vi "Update Fan Status.vi"(8 "error in (no error)":cluster{"状态":bool, "代码":i32, "源":string} caption="错误输入（无错误）", 9 "风扇B":T1, 10 "风扇A":T1, 11 "冷却器UI输入":refnum<class "Live User Controller.lvclass">) -> (0 "error out":cluster{"状态":bool, "代码":i32, "源":string} caption="错误输出", 3 "冷却器UI输出":refnum<class "Live User Controller.lvclass">)   [LabVIEW 2015, in "Live User Controller.lvclass"]
doc: "更新用户接口，显示风扇状态。"
uses:
  Live User Controller.lvclass
  Dual Fan/Dual Fan/Fan Info.ctl
  Live User Controller.lvclass/Live User Controller.ctl
  Dual Fan/Dual Fan/Dual Fan.lvclass
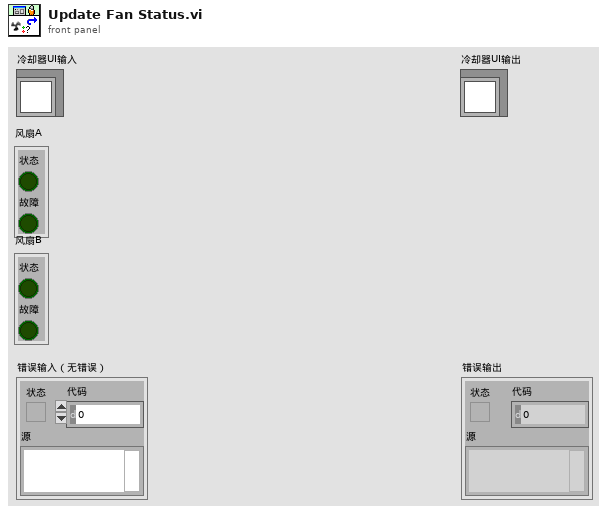
[diagram p1: front panel]
types:
  T1 = typedef "Dual Fan.lvlib/Dual Fan.lvclass/Fan Info.ctl" = cluster{"状态":bool, "故障":bool}
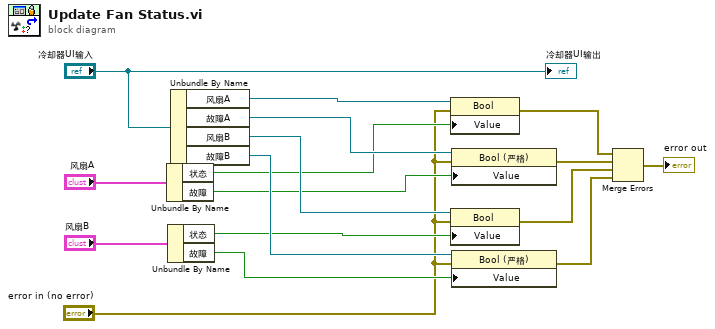
[diagram p0: block diagram]
diagram:
  n1 = Unbundle By Name("风扇A") -> ("状态"=w9:bool, "故障"=w10:bool)
  n2 = Unbundle By Name("风扇B") -> ("状态"=w8:bool, "故障"=w11:bool)
  n3 = Unbundle By Name("冷却器UI输入") -> ("风扇A"=w17:refnum<vi>, "故障A"=w16:refnum<vi>, "风扇B"=w15:refnum<vi>, "故障B"=w14:refnum<vi>)
  n4 = property class="Bool"(reference=w17, error in="error in (no error)", "Value"=w9) -> (error out=w6:errorcluster)  [unwired: 1 out]
  n5 = property class="Bool"(reference=w15, error in="error in (no error)", "Value"=w8) -> (error out=w4:errorcluster)  [unwired: 1 out]
  n6 = property class="Bool (严格)"(reference=w16, error in="error in (no error)", "Value"=w10) -> (error out=w5:errorcluster)  [unwired: 1 out]
  n7 = property class="Bool (严格)"(reference=w14, error in="error in (no error)", "Value"=w11) -> (error out=w3:errorcluster)  [unwired: 1 out]
  n8 = Merge Errors(w6, w5, w4, w3) -> (→"error out":errorcluster)
  "冷却器UI输出" <- "冷却器UI输入"
